vi "Motor Button Setpoint.vi"(8 "Subtract":bool, 9 "ADD":bool, 11 "MotorControlDevRef":T1={"DeviceStatus"={"status"=FALSE, "code"=0, "source"=""}, "Type"=enum."PWM", "PWM"={"Controller"=enum."Controller 1", "PWM Channel"=enum."Invalid", "DeadBand"={"Name"="", "maxPositivePwm"=0, "minPositivePwm"=0, "centerPwm"=0, "maxNegativePwm"=0, "minNegativePwm"=0, "angularRange"=0}}, "CAN"={"Device Number"=0, "Control Mode"=enum."Percent VBus", "Semaphore"=refnum, "Max Vout"=12.0, "TalonSRX Control Mode"=enum."Percent VBus"}, "Invert"=FALSE, "TransformRef"=refnum, "InvTransformRef"=refnum}) -> ()   [LabVIEW 2014]
uses:
  <vilib>/Rock Robotics/WPI/MotorControl/WPI_MotorControlDeviceRef.ctl
  <vilib>/Rock Robotics/WPI/MotorControl/WPI_MotorControlType.ctl
  <vilib>/Rock Robotics/SystemInterfaces/Typedef/FPGA_TypedefDigitalModule.ctl
  <vilib>/Rock Robotics/SystemInterfaces/DIO/FPGA_DIOPWMChannel.ctl
  <vilib>/Rock Robotics/WPI/PWM/WPI_PWMDeadband.ctl
  <vilib>/Rock Robotics/WPI/CAN/Jaguar/SubVIs/WPI_CANJaguar_ControlMode.ctl
  <vilib>/Rock Robotics/WPI/CAN/TalonSRX/WPI_CANTalonSRX_APIControlMode.ctl
  <vilib>/Rock Robotics/WPI/PWM/WPI_PWMTransform_ConPane.ctl
panel:
  in  "Speed":dbl
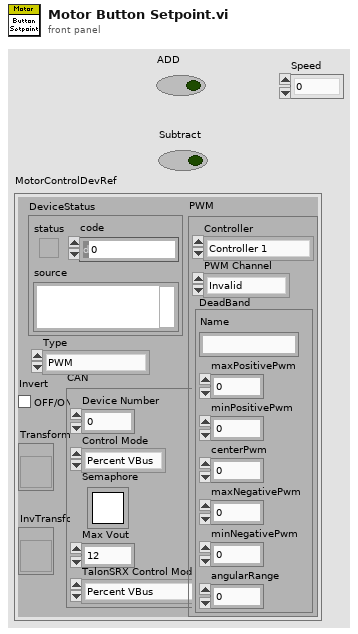
[diagram p1: front panel]
types:
  T1 = typedef "WPI_MotorControlDeviceRef.ctl" = cluster{"DeviceStatus":errorcluster, "Type":T2, "PWM":cluster{"Controller":T3, "PWM Channel":T4, "DeadBand":T5}, "CAN":cluster{"Device Number":u8, "Control Mode":T6, "Semaphore":T7, "Max Vout":dbl, "TalonSRX Control Mode":T8}, "Invert":bool, "TransformRef":T9, "InvTransformRef":T9}
  T2 = typedef "WPI_MotorControlType.ctl" = enum16{"PWM", "CAN", "CANTalonSRX"}
  T3 = typedef "FPGA_TypedefDigitalModule.ctl" = enum16{"Controller 1"}
  T4 = typedef "FPGA_DIOPWMChannel.ctl" = enum8{"PWM 0", "PWM 1", "PWM 2", "PWM 3", "PWM 4", "PWM 5", "PWM 6", "PWM 7", "PWM 8", "PWM 9", "PWM MXP 0", "PWM MXP 1", "PWM MXP 2", "PWM MXP 3", "PWM MXP 4", "PWM MXP 5", "PWM MXP 6", "PWM MXP 7", "PWM MXP 8", "PWM MXP 9", "Invalid"}
  T5 = typedef "WPI_PWMDeadband.ctl" = cluster{"Name":string, "maxPositivePwm":i32, "minPositivePwm":i32, "centerPwm":i32, "maxNegativePwm":i32, "minNegativePwm":i32, "angularRange":u16}
  T6 = typedef "WPI_CANJaguar_ControlMode.ctl" = enum8{"Percent VBus", "Current", "Speed", "Position", "Voltage"}
  T7 = typedef "Semaphore RefNum" = refnum<k1>
  T8 = typedef "WPI_CANTalonSRX_APIControlMode.ctl" = enum8{"Percent VBus", "Speed", "Position", "Slave", "Unchanged / Invalid"}
  T9 = typedef "WPI_PWMTransform_ConPane.ctl" = refnum<vi>
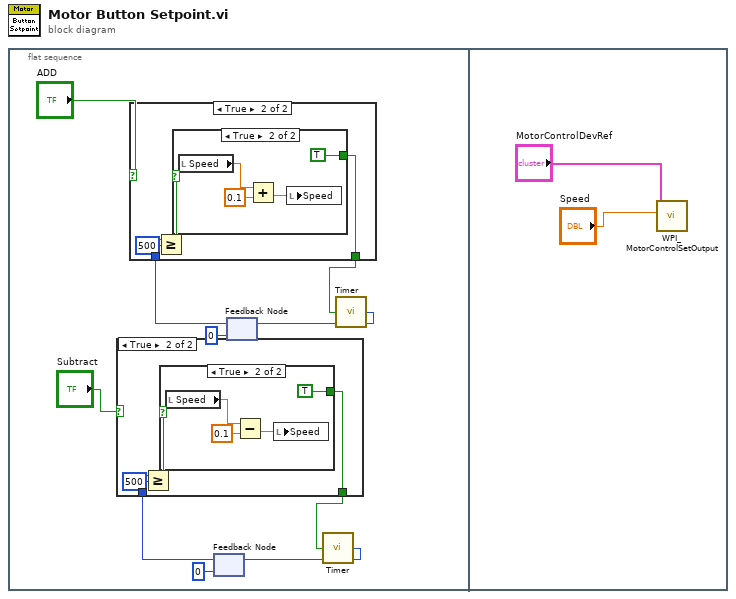
[diagram p0: block diagram]
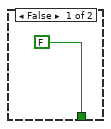
[diagram p2: hidden frame]
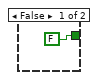
[diagram p3: hidden frame]
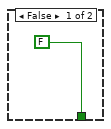
[diagram p4: hidden frame]
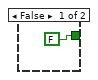
[diagram p5: hidden frame]
diagram:
  n1 = flat-sequence {
    frame #0 {
      n2 = feedback #1(u64 0 ("Time elapsed")) -> (w8:u64)
      n3 = case shown="True" "Subtract" {
        tunnel: [FALSE w15] -> w6
        tunnel: w8 -> [_ w14]
        frame False {
        }
        frame True {
          n4 = Greater Or Equal?(x=w14, y=u64 500) -> (x >= y?=w12:bool)
          n5 = case shown="True" w12 {
            tunnel: [FALSE TRUE] -> w15
            frame False {
            }
            frame True {
              n6 = local read "Speed"() -> (w20:dbl)
              n7 = Subtract(x=w20, y=0.1) -> (x-y=w19:dbl)
              n8 = local write "Speed"(w19) -> ()
            }
          }
        }
      }
      n9 = feedback #2(u64 0 ("Time elapsed")) -> (w4:u64)
      n10 = case shown="True" "ADD" {
        tunnel: [FALSE w25] -> w2
        tunnel: w4 -> [_ w24]
        frame False {
        }
        frame True {
          n11 = Greater Or Equal?(x=w24, y=u64 500) -> (x >= y?=w22:bool)
          n12 = case shown="True" w22 {
            tunnel: [FALSE TRUE] -> w25
            frame False {
            }
            frame True {
              n13 = local read "Speed"() -> (w30:dbl)
              n14 = Add(x=w30, y=0.1) -> (x+y=w28:dbl)
              n15 = local write "Speed"(w28) -> ()
            }
          }
        }
      }
      n16 = call "Timer.vi"("Set Timer"=w6) -> ("Time elapsed"=w7:u64)
      n17 = feedback-in #1(w7) -> ()
      n18 = call "Timer.vi"("Set Timer"=w2) -> ("Time elapsed"=w3:u64)
      n19 = feedback-in #2(w3) -> ()
    }
    frame #1 {
      n20 = call <vilib>:"WPI_MotorControlSetOutput.vi"("Output"="Speed", "MotorControlDevRef"="MotorControlDevRef") -> ()  [unwired: 7 in, 3 out]
    }
  }
